vi "题目二.vi"() -> ()   [LabVIEW 2017]
panel:
  out "和2":i32
  out "和1":i32
  out "数值":i32
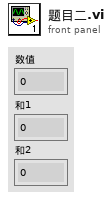
[diagram p1: front panel]
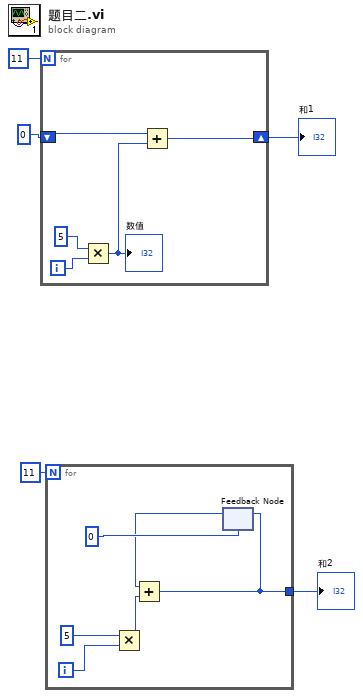
[diagram p0: block diagram]
diagram:
  n1 = for {
    N: 11 -> [_]
    shift-right: [w6] -> w2
    shift-left: 0 -> [w7]
    i -> [w10]
    n2 = Multiply(x=5, y=w10) -> (x*y=w8:i32)
    "数值" <- w8
    n3 = Add(x=w7, y=w8) -> (x+y=w6:i32)
  }
  "和1" <- w2
  n4 = for {
    N: 11 -> [_]
    tunnel: [w11] -> w1
    i -> [w16]
    n5 = Multiply(x=5, y=w16) -> (x*y=w14:i32)
    n6 = feedback #1(0) -> (w12:i32)
    n7 = Add(x=w12, y=w14) -> (x+y=w11:i32)
    n8 = feedback-in #1(w11) -> ()
  }
  "和2" <- w1
